vi "Get Result Section Refs.vi"(8 "Error in":errorcluster, 11 "Device Ref in":T1 format="%.0x") -> (0 "Error out":errorcluster, 2 "Result Section Refs":T1[](array[typedef]) format="%.0x", 3 "Device Ref out":T1 format="%.0x")   [LabVIEW 2014, in "Waveform-Processing-Custom-Device System Explorer.lvlib"]
uses:
  Waveform-Processing-Custom-Device System Explorer.lvlib
  <vilib>/NI Veristand/Custom Device API/Custom Device Item Ref.ctl
  Shared/Constants.vi
  <vilib>/NI Veristand/Custom Device Tools/Custom Device Utility Library/NI VeriStand - Search for All Items by GUID.vi
  <vilib>/NI Veristand/Custom Device Tools/Custom Device Utility Library/Custom Device Utility Library.lvlib
  Shared/Waveform-Processing-Custom-Device Shared.lvlib
  <vilib>/NI Veristand/Custom Device API/Custom Device API.lvlib
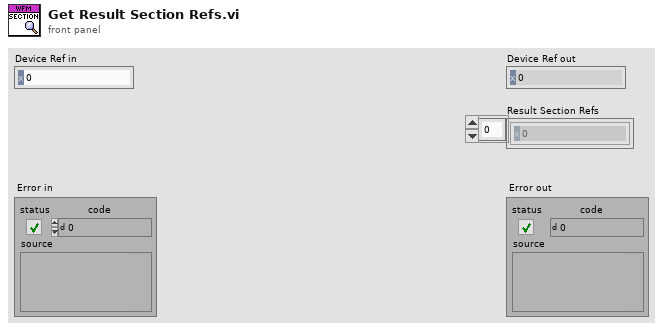
[diagram p1: front panel]
types:
  T1 = typedef "Custom Device API.lvlib/Custom Device Item Ref.ctl" = u64
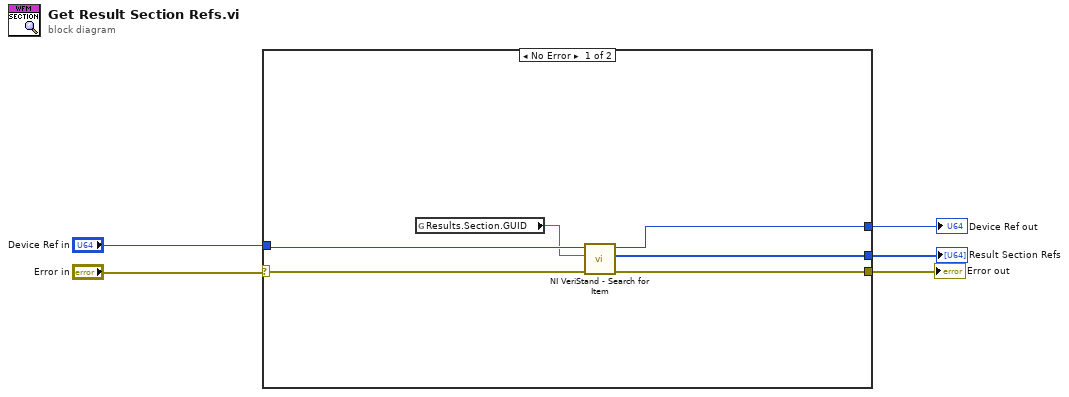
[diagram p0: block diagram]
diagram:
  n1 = case shown="No Error" "Error in" {
    selector: "Error in" -> [w11 w13]
    tunnel: [w8 w13] -> w4
    tunnel: "Device Ref in" -> [w10 w12]
    tunnel: [w7 _] -> w2
    tunnel: [w6 w12] -> w1
    frame No Error {
      n2 = global read "Constants.vi" "Results.Section.GUID"() -> (w9:string)
      n3 = call-poly <vilib>:"NI VeriStand - Search for Item.vi"("error in"=w11, "Item GUID"=w9, "Section Ref in"=w10) -> ("error out"=w8:errorcluster, "Item Refs"=w7:T1[], "Section Ref out"=w6:T1)  [unwired: 5 in, 1 out]
    }
    frame Error {
    }
  }
  "Error out" <- w4
  "Result Section Refs" <- w2
  "Device Ref out" <- w1
